vi "To JSON.vi"(6 "Pretty Print?":bool, 8 "error in (no error)":errorcluster, 11 "Double Float in":refnum<class "Abs_Complex Extended Float.lvclass">) -> (0 "error out":errorcluster, 2 "JSON":string, 3 "Double Float out":refnum<class "Abs_Complex Extended Float.lvclass">)   [LabVIEW 2021, in "Abs_Complex Extended Float.lvclass"]
uses:
  Abs_Complex Extended Float.lvclass
  C:/Program Files (x86)/National Instruments/LabVIEW 2021/vi.lib/TSA/Abstract Data Classes/Abs_Types/Type/Abs_Type.lvclass
  a532f5bb-072c-4b72-b216-7c0fab5fcf4d.vi
  <vilib>/Utility/LVClass/Get LV Class Name.vi
  <vilib>/JDP Science/JSONtext/Variant to JSON Text.vi
  <vilib>/JDP Science/JSONtext/Set Multiple Object Items.vi
  <vilib>/JDP Science/JSONtext/LVClass Serializer/JSONtext LVClass Serializer.lvclass
  Floating Point/Abs_Floating Point.lvclass
  Type/Abs_Type.lvclass
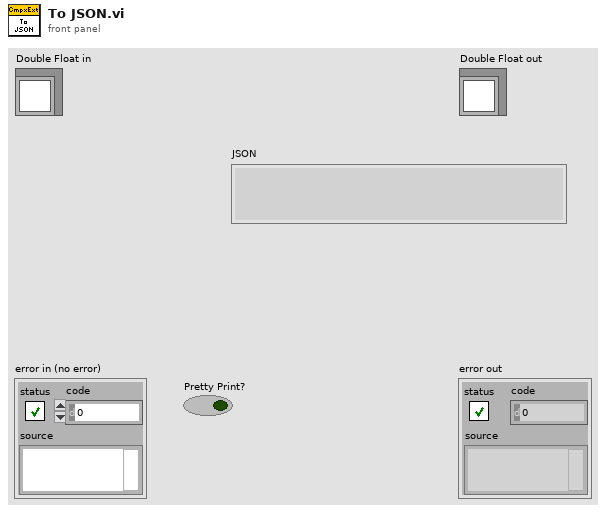
[diagram p1: front panel]
types:
  T1 = typedef "Abs_Complex Extended Float.lvclass/Type.ctl" = cxt
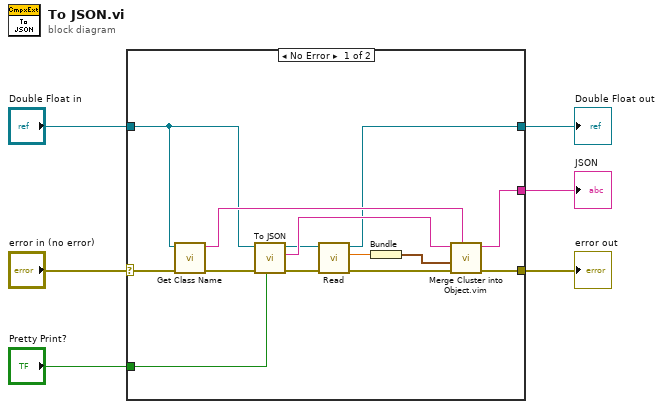
[diagram p0: block diagram]
diagram:
  n1 = case shown="No Error" "error in (no error)" {
    selector: "error in (no error)" -> [w14 w22]
    tunnel: "Double Float in" -> [w8 w21]
    tunnel: [w10 w21] -> w4
    tunnel: [w19 w22] -> w2
    tunnel: [w18 _] -> w3
    tunnel: "Pretty Print?" -> [w7 _]
    frame No Error {
      n2 = call "Get Class Name.vi"("error in (no error)"=w14, "Abs_Type in"=w8) -> ("error out"=w13:errorcluster, "class name"=w16:string)  [unwired: 8 in]
      n3 = call-parent "To JSON.vi"("Pretty Print?"=w7, "error in (no error)"=w13, "Type in"=w8) -> ("error out"=w12:errorcluster, "JSON"=w15:string, "Type out"=w9:refnum<class "Abs_Complex Extended Float.lvclass">)  [unwired: 6 in]
      n4 = call-dynamic "Read.vi"("error in (no error)"=w12, "Double Float.lvclass_340760 in"=w9) -> ("error out"=w11:errorcluster, "Value"=w17:T1, "Double Float.lvclass_340760 out"=w10:refnum<class "Abs_Complex Extended Float.lvclass">)  [unwired: 7 in]
      n5 = Bundle("Value"=w17) -> (w20:cluster{"Value":T1})  [unwired: 1 in]
      n6 = call "Merge Cluster into Object.vim"("$Path or Item Name"=w16, "error in (no error)"=w11, "Any Cluster"=w20, "JSON"=w15) -> ("error out"=w19:errorcluster, "<JSON>"=w18:string)  [unwired: 5 in]
    }
    frame Error {
    }
  }
  "error out" <- w2
  "Double Float out" <- w4
  "JSON" <- w3
